vi "Display Output.vi"(8 "error in (no error)":errorcluster, 10 "Timeout (2000ms)":u32=2000, 11 "VISA resource name":refnum<visa-resource-name>) -> (0 "error out":errorcluster, 1 "Block Data":string, 2 "Read Data":string, 3 "VISA resource name out":refnum<visa-resource-name>)   [LabVIEW 2009, in "DSO1K.lvlib"]
doc: "This VI returns the current screen for RGB 16Bit RLE (Run-Length Encoding) graphic data."
uses:
  <instrlib>/DSO1K/DSO1K.lvlib
  <vilib>/Instr/_visa.llb/VISA Set IO Buffer Mask.ctl
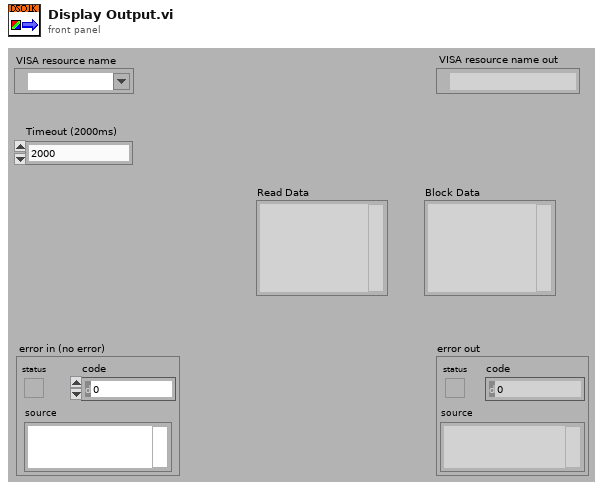
[diagram p1: front panel]
types:
  T1 = typedef "VISA Set IO Buffer Mask.ctl" = u16
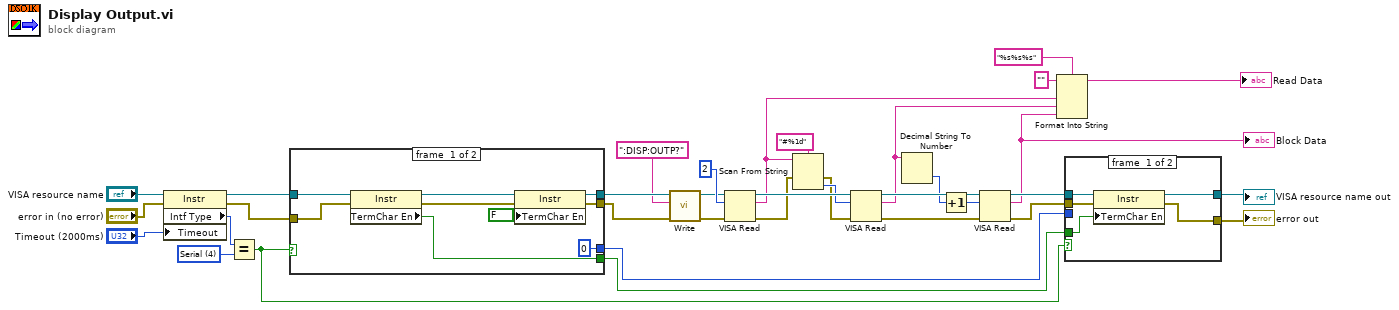
[diagram p0: block diagram]
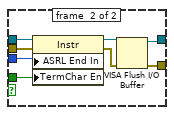
[diagram p2: hidden frame]
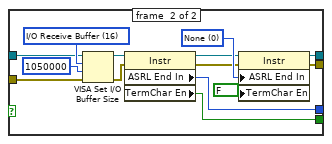
[diagram p3: hidden frame]
diagram:
  w26 = u16 4 items=["GPIB"=1, "VXI"=2, "GPIB-VXI"=3, "Serial"=4, "PXI"=5, "TCPIP"=6, "USB"=7, "FireWire"=9] ("Interface Information:Interface Type")
  n1 = property class="Instr"(reference="VISA resource name", error in="error in (no error)", "Timeout"="Timeout (2000ms)") -> (reference out=w27:refnum<visa-resource-name>, error out=w28:errorcluster, "Intf Type"=w29:u16)
  n2 = Equal?(x=w29, y=w26) -> (x = y?=w23:bool)
  n3 = case shown="True" w23 {
    tunnel: w27 -> [w37 w46]
    tunnel: w28 -> [w36 w45]
    tunnel: [u16 0 ("ASRL End In") w55] -> w25
    tunnel: [w40 w54] -> w13
    tunnel: [w39 w53] -> w11
    tunnel: [w41 w51] -> w24
    frame #0 {
      n4 = property class="Instr"(reference=w37, error in=w36) -> (reference out=w43:refnum<visa-resource-name>, error out=w42:errorcluster, "TermChar En"=w41:bool)
      n5 = property class="Instr"(reference=w43, error in=w42, "TermChar En"=FALSE ("Message Based Settings:Termination Character Enable")) -> (reference out=w40:refnum<visa-resource-name>, error out=w39:errorcluster)
    }
    frame #1 {
      w47 = T1 16 items=["I/O Receive Buffer"=16, "I/O Transmit Buffer"=32, "I/O Receive and Transmit Buffer"=48] ("Mask")
      w58 = u16 0 items=["None", "Last Bit", "TermChar"] ("Serial Settings:End Mode for Reads")
      n6 = VISA Set I/O Buffer Size(VISA resource name=w46, mask (16)=w47, size (4096)=u32 1050000 ("Receive Buffer (4096)"), error in (no error)=w45) -> (VISA resource name out=w50:refnum<visa-resource-name>, error out=w49:errorcluster)
      n7 = property class="Instr"(reference=w50, error in=w49) -> (reference out=w57:refnum<visa-resource-name>, error out=w56:errorcluster, "ASRL End In"=w55:u16, "TermChar En"=w51:bool)
      n8 = property class="Instr"(reference=w57, error in=w56, "ASRL End In"=w58, "TermChar En"=FALSE) -> (reference out=w54:refnum<visa-resource-name>, error out=w53:errorcluster)
    }
  }
  n9 = call <instrlib>:"Write.vi"("error in (no error)"=w11, "Write Buffer (\"\")"=":DISP:OUTP?" ("write buffer"), "VISA resource name"=w13) -> ("error out"=w10:errorcluster, "VISA resource name out"=w12:refnum<visa-resource-name>)  [unwired: 6 in, 1 out]
  n10 = VISA Read(VISA resource name=w12, byte count=u32 2, error in (no error)=w10) -> (VISA resource name out=w33:refnum<visa-resource-name>, read buffer=w6:string, error out=w15:errorcluster)  [unwired: 1 out]
  n11 = Scan From String(format string="#%1d", input string=w6, error in=w15) -> (error out=w14:errorcluster, output 1=w32:i32)  [unwired: 2 in, 2 out]
  n12 = VISA Read(VISA resource name=w33, byte count=w32, error in (no error)=w14) -> (VISA resource name out=w31:refnum<visa-resource-name>, read buffer=w5:string, error out=w30:errorcluster)  [unwired: 1 out]
  n13 = Decimal String To Number(string=w5) -> (number=w7:i32)  [unwired: 2 in, 1 out]
  n14 = Increment(x=w7) -> (x+1=w8:i32)
  n15 = VISA Read(VISA resource name=w31, byte count=w8, error in (no error)=w30) -> (VISA resource name out=w21:refnum<visa-resource-name>, read buffer=w4:string, error out=w20:errorcluster)  [unwired: 1 out]
  "Block Data" <- w4
  n16 = Format Into String(format string="%s%s%s", initial string="", w6, w5, w4) -> (resulting string=→"Read Data":string)  [unwired: 1 in, 1 out]
  n17 = case shown="True" w23 {
    tunnel: [w63 w67] -> w18
    tunnel: [w62 w66] -> w17
    tunnel: w21 -> [w61 w71]
    tunnel: w20 -> [w60 w70]
    tunnel: w25 -> [_ w65]
    tunnel: w24 -> [w59 w64]
    frame #0 {
      n18 = property class="Instr"(reference=w61, error in=w60, "TermChar En"=w59) -> (reference out=w63:refnum<visa-resource-name>, error out=w62:errorcluster)
    }
    frame #1 {
      n19 = property class="Instr"(reference=w71, error in=w70, "ASRL End In"=w65, "TermChar En"=w64) -> (reference out=w69:refnum<visa-resource-name>, error out=w68:errorcluster)
      n20 = VISA Flush I/O Buffer(VISA resource name=w69, error in (no error)=w68) -> (VISA resource name out=w67:refnum<visa-resource-name>, error out=w66:errorcluster)  [unwired: 1 in]
    }
  }
  "error out" <- w17
  "VISA resource name out" <- w18
